vi "front_panel.vi"() -> ()   [LabVIEW 2020]
uses:
  Enum State Control.ctl
  <vilib>/numeric/Random Number (Range) U64.vi
  <vilib>/numeric/sub_Random U32.vi
panel:
  in  "boom":u16(ring)
  in  "Tab Control":enum32{"Game", " Ranking"}(tab)
  in  "Start game":bool
  out "START":bool
  in  "Right":bool
  in  "Left":bool
  out "Time":dbl
  out "Points":u32
  out "Level":u8
  in  "stop":bool
  in  "Spacecraft":u16(ring)
  in  "Alien":u16(ring)
  out "Shot":bool
  out "Life":u8(slide) scale=0.0..3.0
  in  "Shoot":bool
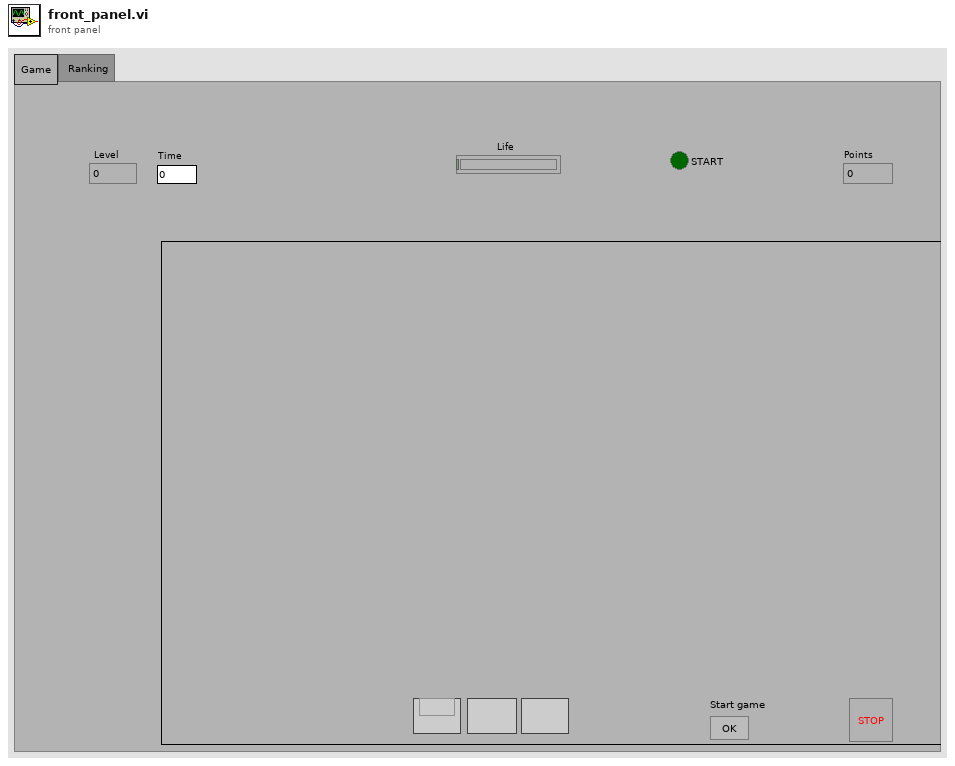
[diagram p1: front panel]
types:
  T1 = typedef "Enum State Control.ctl" = enum16{"Init", "Start ", "Stop", "Left", "Right"}
  T2 = typedef "LVPositionTypeDef.ctl" = cluster{"Left":i32, "Top":i32}
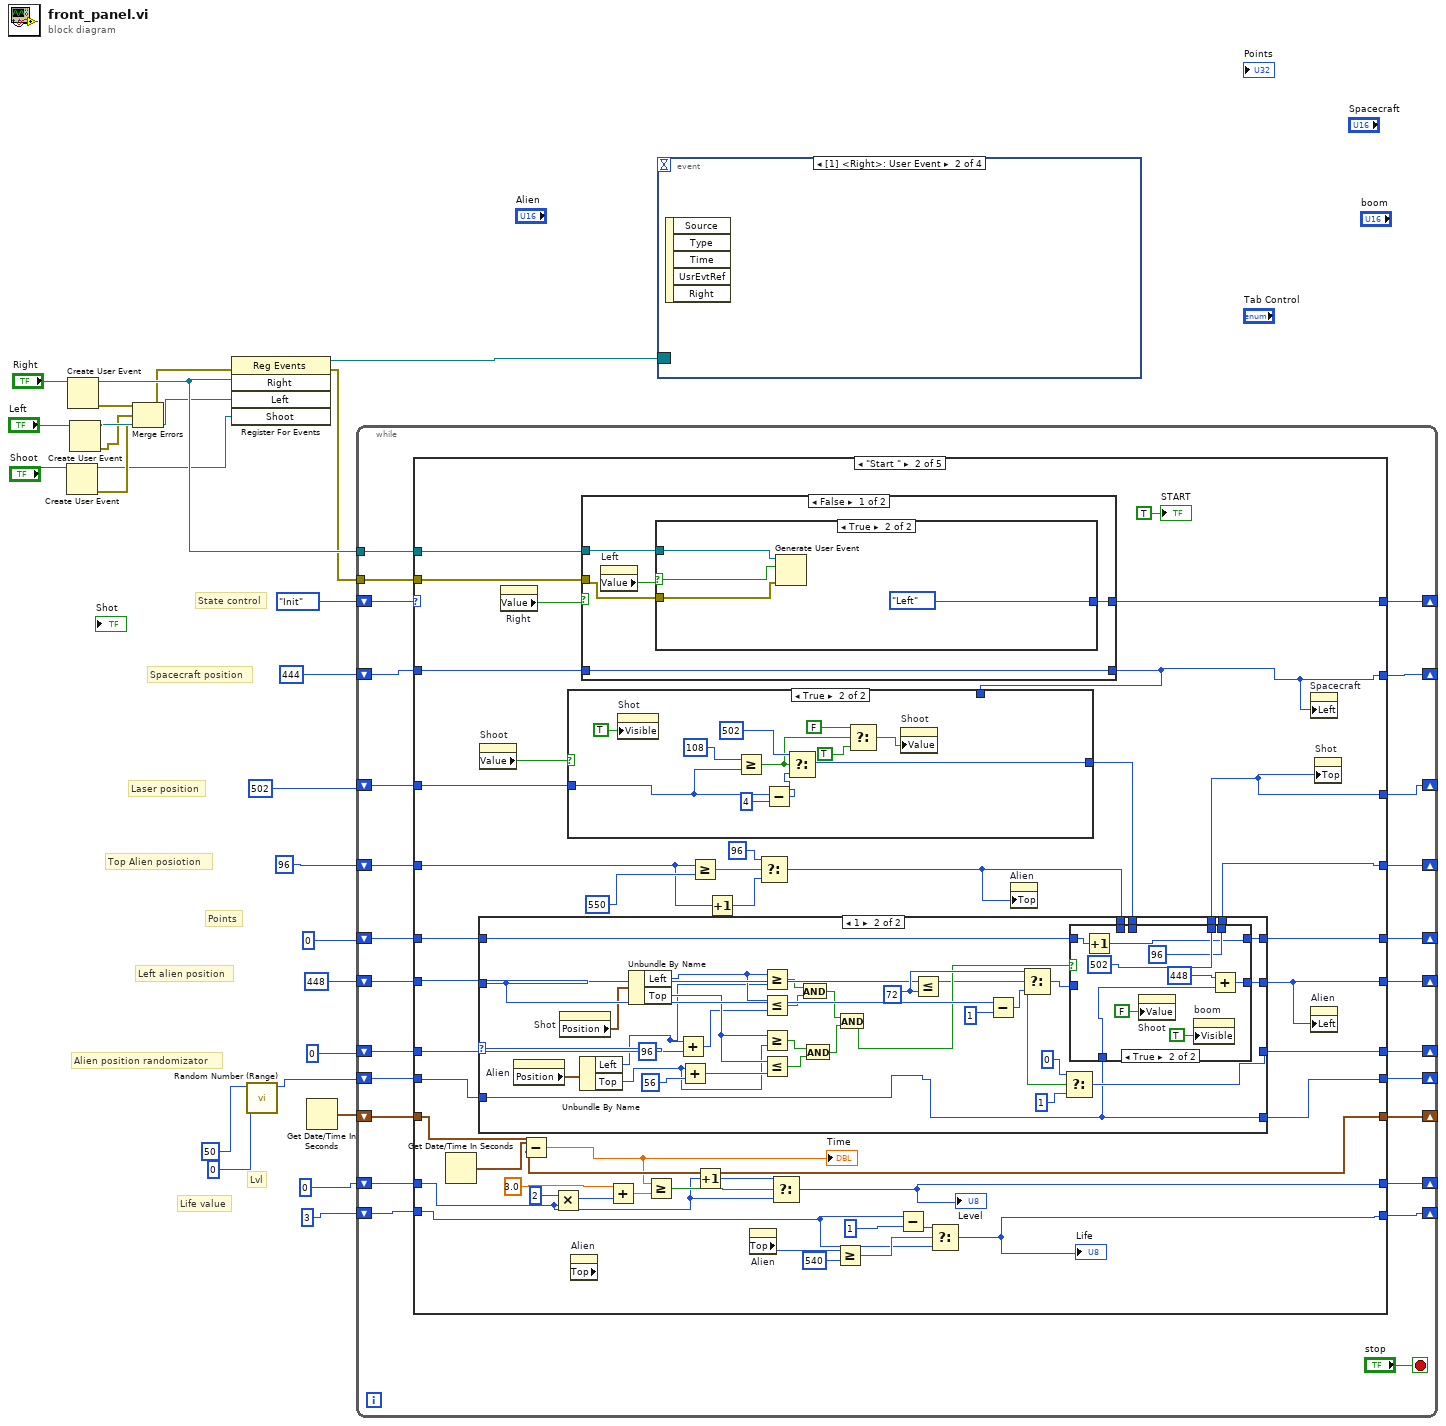
[diagram p0: block diagram]
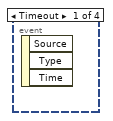
[diagram p2: hidden frame]
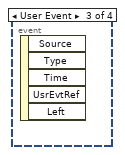
[diagram p3: hidden frame]
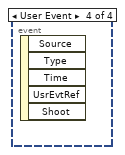
[diagram p4: hidden frame]
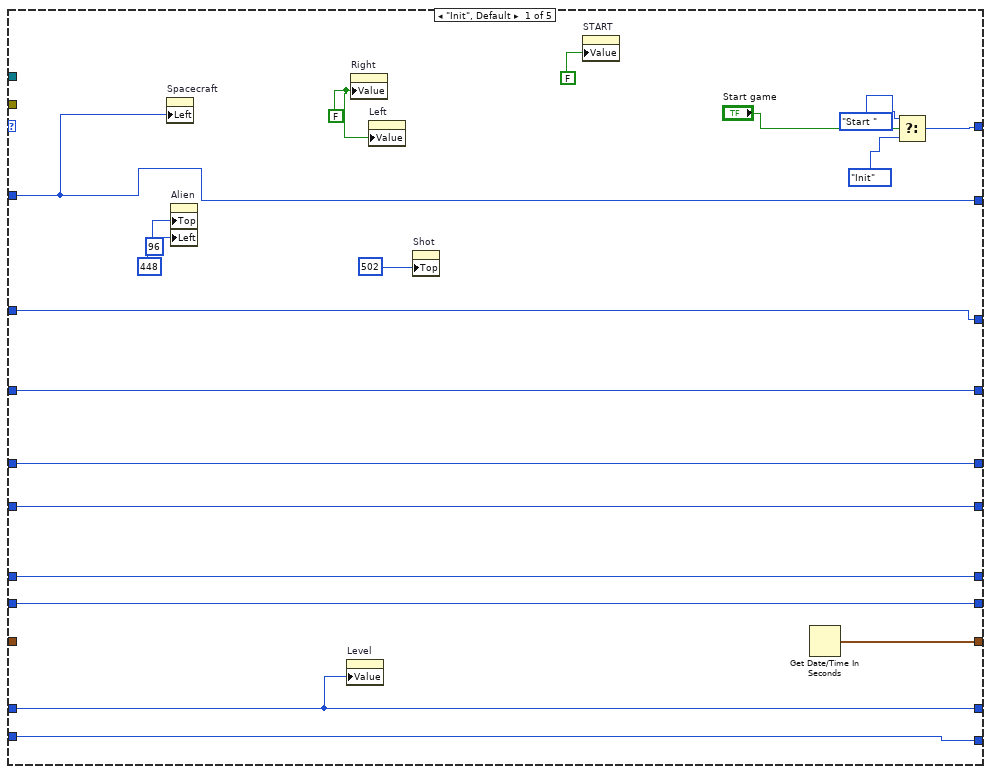
[diagram p5: hidden frame]
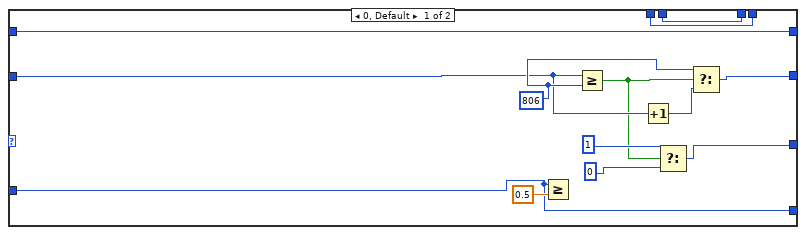
[diagram p6: hidden frame]
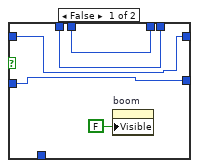
[diagram p7: hidden frame]
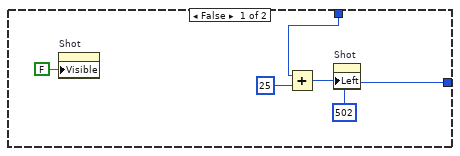
[diagram p8: hidden frame]
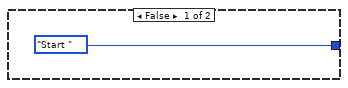
[diagram p9: hidden frame]
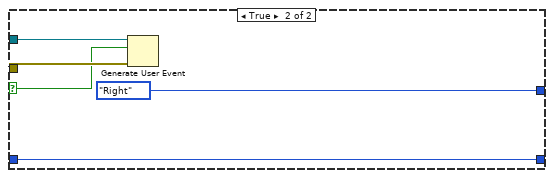
[diagram p10: hidden frame]
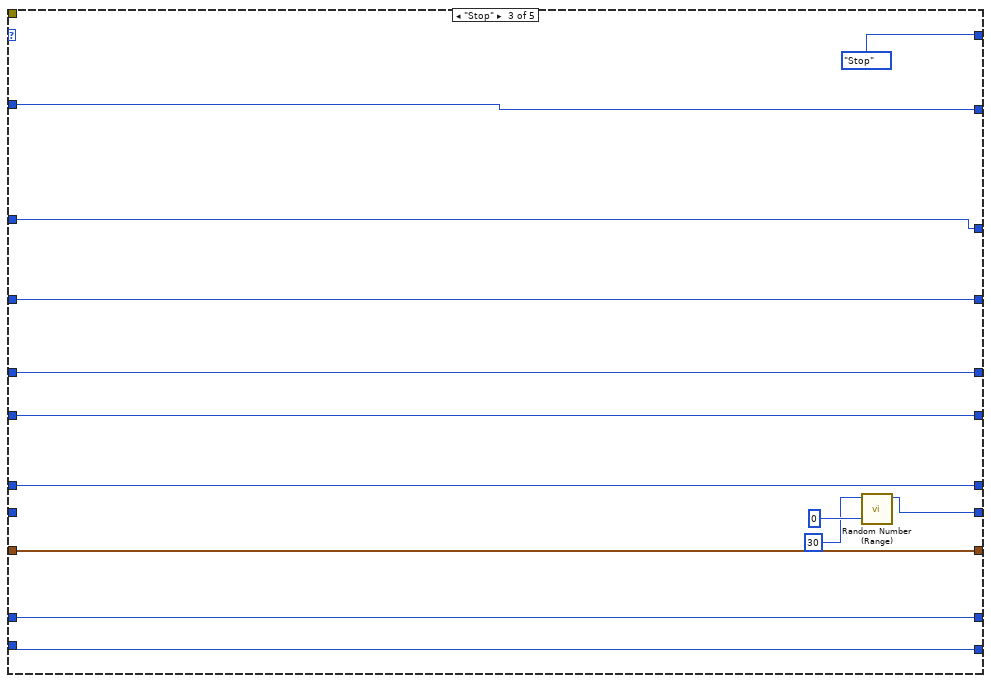
[diagram p11: hidden frame]
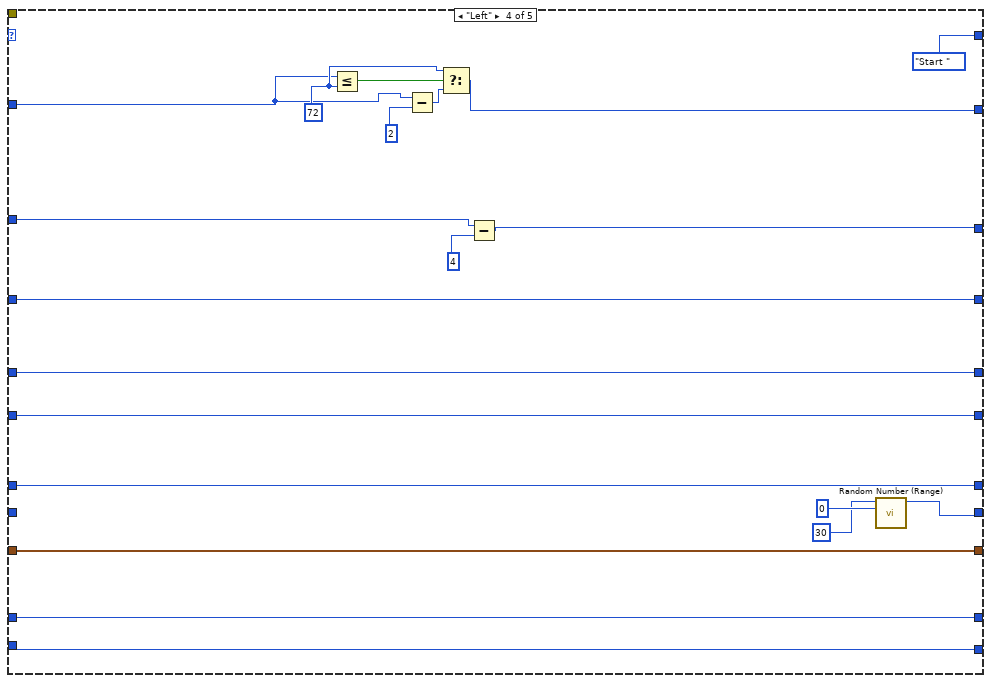
[diagram p12: hidden frame]
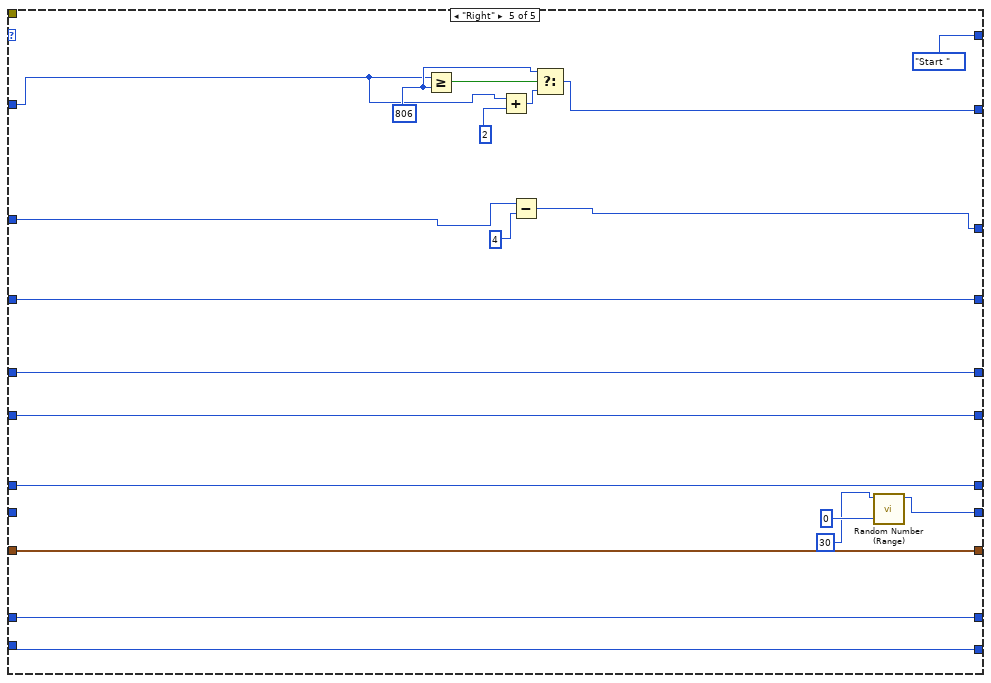
[diagram p13: hidden frame]
diagram:
  # "Points"
  # "Lvl"
  # "Life value"
  # "Alien position randomizator"
  # "Left alien position"
  # "Top Alien posiotion"
  # "Laser position"
  # "Spacecraft position"
  # "State control"
  n1 = Create User Event(user event datatype="Shoot") -> (user event=w12:refnum<user-event>, error out=w13:errorcluster)  [unwired: 1 in]
  n2 = Create User Event(user event datatype="Right") -> (user event=w22:refnum<user-event>, error out=w17:errorcluster)  [unwired: 1 in]
  n3 = Create User Event(user event datatype="Left") -> (user event=w18:refnum<user-event>, error out=w16:errorcluster)  [unwired: 1 in]
  n4 = Merge Errors(w17, w16, w13) -> (w15:errorcluster)
  n5 = register-events(error in=w15, w22, w18, w12) -> (reference out=w23:refnum<event-registration>, error out=w21:errorcluster)  [unwired: 1 in]
  n6 = call-poly <vilib>:"Random Number (Range).vi"("lower bound (0)"=u64 0, "upper bound (100)"=u64 50) -> ("number"=w4:u64)  [unwired: 9 in]
  n7 = Get Date/Time In Seconds() -> (seconds since 1Jan1904=w7:timestamp)
  n8 = while {
    tunnel: w22 -> [w48]
    shift-right: [w47] -> _
    shift-left: Enum_State_Control."Init" -> [w49]
    tunnel: w21 -> [w46]
    shift-right: [w44] -> _
    shift-left: 444 ("Position:Left") -> [w45]
    shift-right: [w42] -> _
    shift-left: 502 ("y") -> [w43]
    shift-right: [w40] -> _
    shift-left: 96 ("Position:Top") -> [w41]
    shift-right: [w39] -> _
    shift-left: 448 ("Position:Left") -> [w38]
    shift-right: [w37] -> _
    shift-left: 0 -> [w36]
    shift-right: [w35] -> _
    shift-left: w7 -> [w34]
    shift-right: [w32] -> _
    shift-left: w4 -> [w33]
    shift-right: [w31] -> _
    shift-left: u8 3 ("Life") -> [w30]
    shift-right: [w28] -> _
    shift-left: 0 -> [w29]
    shift-right: [w26] -> _
    shift-left: 0 -> [w27]
    stop <- "stop" stop-if-true
    n9 = case shown="\"Start \"" w49 {
      tunnel: w48 -> [_ w113 _ _ _]
      tunnel: [w66 w110 Enum_State_Control."Stop" Enum_State_Control."Start " Enum_State_Control."Start "] -> w47
      tunnel: w46 -> [_ w112 _ _ _]
      tunnel: w45 -> [w65 w111 w217 w234 w253]
      tunnel: [w65 w106 w217 w232 w252] -> w44
      tunnel: w43 -> [w61 w105 w216 w227 w247]
      tunnel: [w61 w95 w216 w226 w246] -> w42
      tunnel: w41 -> [w59 w100 w215 w229 w249]
      tunnel: [w59 w96 w215 w229 w249] -> w40
      tunnel: [w58 w93 w214 w231 w251] -> w39
      tunnel: w38 -> [w58 w99 w214 w231 w251]
      tunnel: [w57 w97 w213 w230 w250] -> w37
      tunnel: w36 -> [w57 w98 w213 w230 w250]
      tunnel: [w56 w91 w212 w225 w245] -> w35
      tunnel: w34 -> [_ w91 w212 w225 w245]
      tunnel: w33 -> [w54 w89 _ _ _]
      tunnel: [w54 w88 w210 w223 w242] -> w32
      tunnel: [w53 w81 w208 w221 w241] -> w31
      tunnel: w30 -> [w53 w83 w208 w221 w241]
      tunnel: w29 -> [w52 w74 w207 w220 w240]
      tunnel: [w52 w79 w207 w220 w240] -> w28
      tunnel: w27 -> [w51 w71 w206 w219 w239]
      tunnel: [w51 w70 w206 w219 w239] -> w26
      frame "Init", Default {
        w63 = FALSE ("Right")
        n10 = property on="Spacecraft" class="Ring (strict)"("Left"=w65) -> ()  [unwired: 2 in, 2 out]
        n11 = property on="Alien" class="Ring (strict)"("Top"=96 ("Position:Top"), "Left"=448 ("Position:Left")) -> ()  [unwired: 2 in, 2 out]
        n12 = property on="Level" class="DigNum (strict)"("Value"=w52) -> ()  [unwired: 2 in, 2 out]
        n13 = property on="Right" class="Bool (strict)"("Value"=w63) -> ()  [unwired: 2 in, 2 out]
        n14 = property on="Left" class="Bool (strict)"("Value"=w63) -> ()  [unwired: 2 in, 2 out]
        n15 = property on="Shot" class="Bool (strict)"("Top"=502 ("y")) -> ()  [unwired: 2 in, 2 out]
        n16 = property on="START" class="Bool (strict)"("Value"=FALSE ("START")) -> ()  [unwired: 2 in, 2 out]
        n17 = Get Date/Time In Seconds() -> (seconds since 1Jan1904=w56:timestamp)
        n18 = Select(t=Enum_State_Control."Start ", s="Start game", f=Enum_State_Control."Init") -> (s? t:f=w66:T1)
      }
      frame "Start " {
        n19 = Get Date/Time In Seconds() -> (seconds since 1Jan1904=w90:timestamp)
        n20 = property on="Shoot" class="Bool (strict)"() -> ("Value"=w107:bool)  [unwired: 2 in, 2 out]
        n21 = property on="Right" class="Bool (strict)"() -> ("Value"=w109:bool)  [unwired: 2 in, 2 out]
        n22 = Subtract(x=w90, y=w91) -> (x-y=w80:dbl)
        "Time" <- w80
        n23 = Multiply(x=2, y=w74) -> (x*y=w75:i32)
        n24 = property on="Alien" class="Ring (strict)" props=["Top"]() -> ()  [unwired: 2 in, 3 out]
        n25 = case shown="False" w109 {
          selector: w109 -> [_ w203]
          tunnel: w113 -> [w193 w205]
          tunnel: w112 -> [w192 w204]
          tunnel: w111 -> [w191 w202]
          tunnel: [w191 w202] -> w106
          tunnel: [w194 Enum_State_Control."Right"] -> w110
          frame False {
            n26 = property on="Left" class="Bool (strict)"() -> ("Value"=w195:bool)  [unwired: 2 in, 2 out]
            n27 = case shown="True" w195 {
              selector: w195 -> [_ w197]
              tunnel: [Enum_State_Control."Start " Enum_State_Control."Left"] -> w194
              tunnel: w193 -> [_ w199]
              tunnel: w192 -> [_ w198]
              frame False {
              }
              frame True {
                n28 = Generate User Event(user event=w199, event data cluster=w197, error in=w198) -> ()  [unwired: 1 in, 2 out]
              }
            }
          }
          frame True {
            n29 = Generate User Event(user event=w205, event data cluster=w203, error in=w204) -> ()  [unwired: 1 in, 2 out]
          }
        }
        n30 = case shown="True" w107 {
          tunnel: w106 -> [w176 _]
          tunnel: w105 -> [_ w182]
          tunnel: [502 ("t") w183] -> w94
          frame False {
            n31 = property on="Shot" class="Bool (strict)"("Visible"=FALSE) -> ()  [unwired: 2 in, 2 out]
            n32 = Add(x=w176, y=25) -> (x+y=w178:i32)
            n33 = property on="Shot" class="Bool (strict)"("Left"=w178) -> ()  [unwired: 2 in, 2 out]
          }
          frame True {
            n34 = property on="Shot" class="Bool (strict)"("Visible"=TRUE) -> ()  [unwired: 2 in, 2 out]
            n35 = Greater Or Equal?(x=108 ("y"), y=w182) -> (x >= y?=w187:bool)
            n36 = Subtract(x=w182, y=4) -> (x-y=w181:i32)
            n37 = Select(t=502, s=w187, f=w181) -> (s? t:f=w183:i32)
            n38 = Select(t=FALSE, s=w187, f=TRUE) -> (s? t:f=w184:bool)
            n39 = property on="Shoot" class="Bool (strict)"("Value"=w184) -> ()  [unwired: 2 in, 2 out]
          }
        }
        n40 = Add(x=3.0 ("y"), y=w75) -> (x+y=w77:dbl)
        n41 = Greater Or Equal?(x=w80, y=w77) -> (x >= y?=w78:bool)
        n42 = Greater Or Equal?(x=w100, y=550) -> (x >= y?=w103:bool)
        n43 = Increment(x=w74) -> (x+1=w76:i32)
        n44 = Increment(x=w100) -> (x+1=w101:i32)
        n45 = property on="Alien" class="Ring (strict)"() -> ("Top"=w87:i32)  [unwired: 2 in, 2 out]
        n46 = Select(t=96 ("y"), s=w103, f=w101) -> (s? t:f=w92:i32)
        n47 = case shown="1" w98 {
          tunnel: w99 -> [w124 w154]
          tunnel: [w123 w136] -> w93
          tunnel: [w120 w155] -> w97
          tunnel: [w119 w135] -> w96
          tunnel: w92 -> [w119 w134]
          tunnel: [w118 w133] -> w95
          tunnel: w94 -> [w118 w132]
          tunnel: w89 -> [w116 w130]
          tunnel: [w116 w130] -> w88
          tunnel: w71 -> [w114 w128]
          tunnel: [w114 w127] -> w70
          frame 0, Default {
            w126 = 806 ("y")
            n48 = Greater Or Equal?(x=w116, y=0.5) -> ()  [unwired: 1 out]
            n49 = Greater Or Equal?(x=w124, y=w126) -> (x >= y?=w115:bool)
            n50 = Increment(x=w124) -> (x+1=w125:u64)
            n51 = Select(t=1 ("y"), s=w115, f=0 ("y")) -> (s? t:f=w120:i32)
            n52 = Select(t=w126, s=w115, f=w125) -> (s? t:f=w123:u64)
          }
          frame 1 {
            w159 = 72 ("y")
            n53 = property on="Alien" class="Ring (strict)"() -> ("Position"=w141:T2)  [unwired: 2 in, 2 out]
            n54 = property on="Shot" class="Bool (strict)"() -> ("Position"=w142:T2)  [unwired: 2 in, 2 out]
            n55 = Unbundle By Name(w141) -> ("Left"=w139:i32, "Top"=w138:i32)
            n56 = Unbundle By Name(w142) -> ("Left"=w152:i32, "Top"=w153:i32)
            n57 = Add(x=w139, y=96) -> (x+y=w151:i32)
            n58 = Add(x=w138, y=56) -> (x+y=w150:i32)
            n59 = Greater Or Equal?(x=w152, y=w139) -> (x >= y?=w144:bool)
            n60 = Less Or Equal?(x=w152, y=w151) -> (x <= y?=w145:bool)
            n61 = Greater Or Equal?(x=w153, y=w138) -> (x >= y?=w146:bool)
            n62 = Less Or Equal?(x=w153, y=w150) -> (x <= y?=w147:bool)
            n63 = And(x=w144, y=w145) -> (x .and. y?=w148:bool)
            n64 = And(x=w146, y=w147) -> (x .and. y?=w149:bool)
            n65 = And(x=w148, y=w149) -> (x .and. y?=w137:bool)
            n66 = Less Or Equal?(x=w154, y=w159) -> (x <= y?=w131:bool)
            n67 = Subtract(x=w154, y=1) -> (x-y=w158:u64)
            n68 = Select(t=w159, s=w131, f=w158) -> (s? t:f=w129:u64)
            n69 = Select(t=0 ("y"), s=w131, f=1 ("y")) -> (s? t:f=w155:i32)
            n70 = case shown="True" w137 {
              tunnel: [w162 w168] -> w136
              tunnel: [w165 96 ("y")] -> w135
              tunnel: w134 -> [w165 _]
              tunnel: [w164 502 ("t")] -> w133
              tunnel: w132 -> [w164 _]
              tunnel: w130 -> [_ w172]
              tunnel: w129 -> [w162 _]
              tunnel: w128 -> [w161 w167]
              tunnel: [w161 w166] -> w127
              frame False {
                n71 = property on="boom" class="Ring (strict)"("Visible"=FALSE) -> ()  [unwired: 2 in, 2 out]
              }
              frame True {
                n72 = Increment(x=w167) -> (x+1=w166:i32)
                n73 = property on="Shoot" class="Bool (strict)"("Value"=FALSE ("Shoot")) -> ()  [unwired: 2 in, 2 out]
                n74 = property on="boom" class="Ring (strict)"("Visible"=TRUE) -> ()  [unwired: 2 in, 2 out]
                n75 = Add(x=448 ("y"), y=w172) -> (x+y=w168:u64)
              }
            }
          }
        }
        n76 = Select(t=w76, s=w78, f=w74) -> (s? t:f=w79:i32)
        "Level" <- w79
        n77 = Greater Or Equal?(x=w87, y=540) -> (x >= y?=w85:bool)
        n78 = Subtract(x=w83, y=u8 1) -> (x-y=w84:u8)
        n79 = Select(t=w84, s=w85, f=w83) -> (s? t:f=w81:u8)
        "Life" <- w81
        n80 = property on="Alien" class="Ring (strict)"("Top"=w92) -> ()  [unwired: 2 in, 2 out]
        n81 = property on="Spacecraft" class="Ring (strict)"("Left"=w106) -> ()  [unwired: 2 in, 2 out]
        n82 = property on="Alien" class="Ring (strict)"("Left"=w93) -> ()  [unwired: 2 in, 2 out]
        n83 = property on="Shot" class="Bool (strict)"("Top"=w95) -> ()  [unwired: 2 in, 2 out]
        "START" <- TRUE ("START")
      }
      frame "Stop" {
        n84 = call-poly <vilib>:"Random Number (Range).vi"("lower bound (0)"=u64 0, "upper bound (100)"=u64 30) -> ("number"=w210:u64)  [unwired: 9 in]
      }
      frame "Left" {
        w235 = 72 ("y")
        n85 = Less Or Equal?(x=w234, y=w235) -> (x <= y?=w236:bool)
        n86 = Subtract(x=w234, y=2) -> (x-y=w233:i32)
        n87 = Select(t=w235, s=w236, f=w233) -> (s? t:f=w232:i32)
        n88 = Subtract(x=w227, y=4) -> (x-y=w226:i32)
        n89 = call-poly <vilib>:"Random Number (Range).vi"("lower bound (0)"=u64 0, "upper bound (100)"=u64 30) -> ("number"=w223:u64)  [unwired: 9 in]
      }
      frame "Right" {
        w255 = 806 ("y")
        n90 = Greater Or Equal?(x=w253, y=w255) -> (x >= y?=w256:bool)
        n91 = Add(x=w253, y=2) -> (x+y=w254:i32)
        n92 = Subtract(x=w247, y=4) -> (x-y=w246:i32)
        n93 = Select(t=w255, s=w256, f=w254) -> (s? t:f=w252:i32)
        n94 = call-poly <vilib>:"Random Number (Range).vi"("lower bound (0)"=u64 0, "upper bound (100)"=u64 30) -> ("number"=w242:u64)  [unwired: 9 in]
      }
    }
  }
  n95 = event shown="[1] <Right>: User Event" {
    selector: w23 -> [_ _ _ _]
    dyn-events: _ -> [_ _ _ _]
    timeout: _ -> [_ _ _ _]
    event Timeout {
      n96 = event-data() -> ()  [unwired: 1 in, 3 out]
    }
    event User Event {
      n97 = event-data() -> ()  [unwired: 1 in, 5 out]
    }
    event User Event {
      n98 = event-data() -> ()  [unwired: 1 in, 5 out]
    }
    event User Event {
      n99 = event-data() -> ()  [unwired: 1 in, 5 out]
    }
  }
